vi "Update base path and daily path globals.vi"(8 "error in":errorcluster, 11 "Base Directory":path) -> (0 "error out":errorcluster, 3 "Base Directory (dupl)":path)   [LabVIEW 2013]
uses:
  Global Variables/General Globals.vi
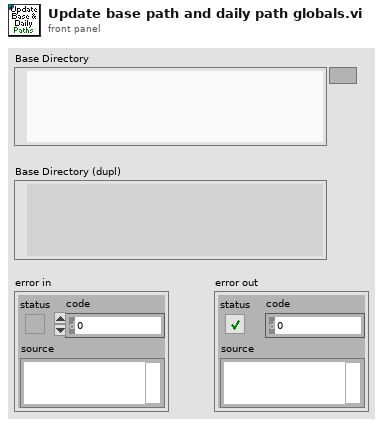
[diagram p1: front panel]
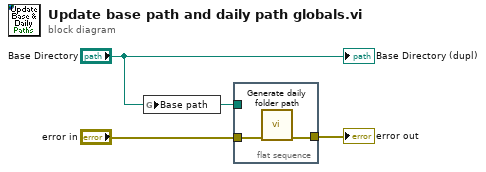
[diagram p0: block diagram]
diagram:
  n1 = global write "General Globals.vi" "Base path"("Base Directory") -> ()
  n2 = flat-sequence {
    tunnel: "Base Directory" -> [_]
    tunnel: [w5] -> w3
    tunnel: "error in" -> [w4]
    frame #0 {
      n3 = call "Generate daily folder path.vi"("error in (no error)"=w4) -> ("error out"=w5:errorcluster)  [unwired: 10 in]
    }
  }
  "error out" <- w3
  "Base Directory (dupl)" <- "Base Directory"
